vi "Actor Core.vi"(8 "error in":errorcluster, 11 "CS++GUIActor in":refnum<class "CS++GUIActor.lvclass">) -> (0 "error out":errorcluster, 3 "Actor out":refnum<class "Actor.lvclass">)   [LabVIEW 2013, in "CS++GUIActor.lvlib" / "CS++GUIActor.lvclass"]
doc: "(<B>Filename</B>: Actor Framework.lvlib:Actor.lvclass:Actor Core.vi)\n\nReceives messages to the actor, reacts to them, and initiates any error handling that may shut the actor down.\n\nDescendant classes may override this VI to append parallel tasks for the actor to complete while it handles messages. Overrides use the Call Parent Method node."
uses:
  CS++GUIActor.lvclass
  <vilib>/ActorFramework/Actor/Actor.lvclass
  CS++BaseActor/CS++BaseActor.lvclass/CS++BaseActor.ctl
  CS++GUIActor.lvclass/CS++GUIActor.ctl
  Classes/CS++BaseClasses/Factory/CS++Factory.lvclass
  CS++BaseActor/CS++BaseActor.lvclass
  <vilib>/ActorFramework/Actor/Actor.lvclass/Actor.ctl
  <vilib>/ActorFramework/Message Enqueuer/Message Enqueuer.lvclass/Message Enqueuer.ctl
  <vilib>/ActorFramework/Message Enqueuer/Init from Existing Queue.vi
  <vilib>/ActorFramework/Message Enqueuer/Enqueue.vi
  <vilib>/ActorFramework/Message Priority Queue/Priority Enqueue.vi
  <vilib>/ActorFramework/Message Enqueuer/Message Enqueuer.lvclass
  <vilib>/ActorFramework/Stop Msg/Stop Msg.lvclass
panel:
  in  "Stop Button":bool
  out "Actor Name":string
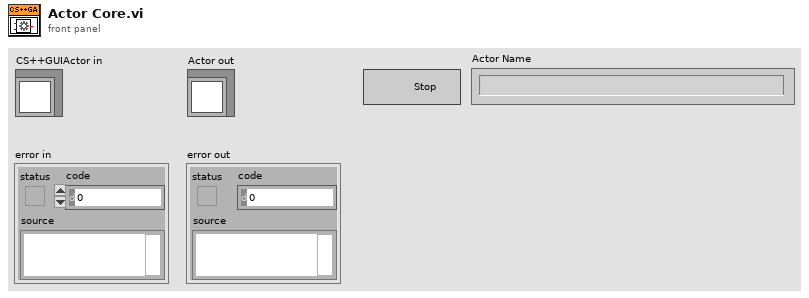
[diagram p1: front panel]
types:
  T1 = enum32{"Invalid", "Standard", "Closed", "Hidden", "Minimized", "Maximized"}
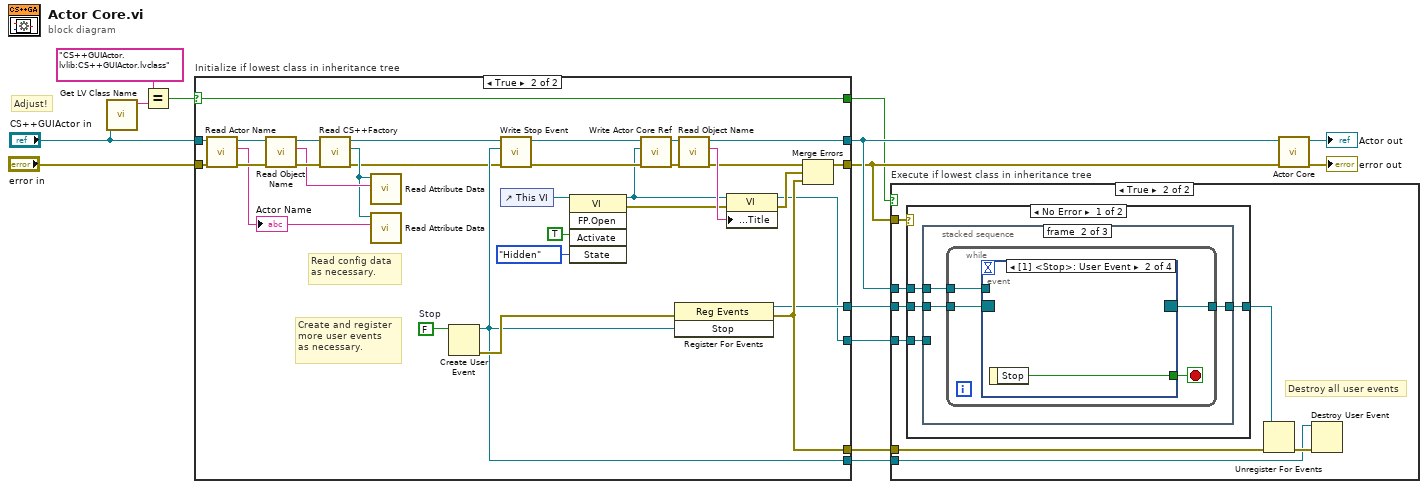
[diagram p0: block diagram]
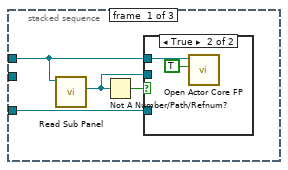
[diagram p3: hidden frame]
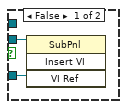
[diagram p4: hidden frame]
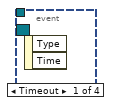
[diagram p5: hidden frame]
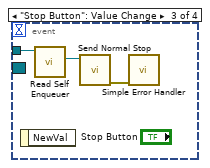
[diagram p6: hidden frame]
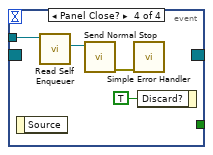
[diagram p7: hidden frame]
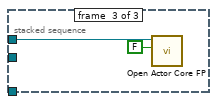
[diagram p8: hidden frame]
diagram:
  # "Adjust!"
  n1 = call <vilib>:"Get LV Class Name.vi"("object"="CS++GUIActor in") -> ("class name"=w13:string)  [unwired: 9 in, 1 out]
  n2 = Equal?(x="CS++GUIActor.lvlib:CS++GUIActor.lvclass" ("class name"), y=w13) -> (x = y?=w2:bool)
  n3 = case "Initialize if lowest class in inheritance tree" shown="True" w2 {
    selector: w2 -> [w17 w20]
    tunnel: "error in" -> [w15 w49]
    tunnel: "CS++GUIActor in" -> [w16 w48]
    tunnel: [_ w40] -> w8
    tunnel: [_ w39] -> w7
    tunnel: [_ w18] -> w6
    tunnel: [_ w30] -> w5
    tunnel: [w16 w22] -> w4
    tunnel: [w15 w21] -> w3
    tunnel: [w17 w20] -> w1
    frame False {
    }
    frame True {
      w43 = FALSE  # Stop
      # "Create and register \nmore user events\nas necessary."
      # "Read config data\nas necessary."
      n4 = call "Read Actor Name.vi"("error in (no error)"=w49, "CS++GUIActor in"=w48) -> ("error out"=w33:errorcluster, "Actor Name"=w31:string, "CS++GUIActor out"=w34:refnum<class "CS++GUIActor.lvclass">)  [unwired: 7 in]
      "Actor Name" <- w31
      n5 = call "Read Object Name.vi"("error in (no error)"=w33, "CS++BaseActor in"=w34) -> ("error out"=w36:errorcluster, "Object Name"=w35:string, "CS++BaseActor out"=w37:refnum<class "CS++GUIActor.lvclass">)  [unwired: 7 in]
      n6 = call "Read CS++Factory.vi"("error in (no error)"=w36, "CS++BaseActor in"=w37) -> ("error out"=w28:errorcluster, "CS++Factory"=w32:refnum<class "CS++Factory.lvclass">, "CS++BaseActor out"=w29:refnum<class "CS++GUIActor.lvclass">)  [unwired: 7 in]
      n7 = call-dynamic "Read Attribute Data.vi"("Object Name"=w35, "CS++Factory in"=w32) -> ()  [unwired: 7 in, 3 out]
      n8 = call-dynamic "Read Attribute Data.vi"("Object Name"=w31, "CS++Factory in"=w32) -> ()  [unwired: 7 in, 3 out]
      n9 = Create User Event(user event datatype=w43) -> (user event=w30:refnum<user-event>, error out=w41:errorcluster)  [unwired: 1 in]
      n10 = call "Write Stop Event.vi"("error in (no error)"=w28, "Stop"=w30, "CS++GUIActor in"=w29) -> ("error out"=w26:errorcluster, "CS++GUIActor out"=w27:refnum<class "CS++GUIActor.lvclass">)  [unwired: 7 in]
      n11 = control-ref of="This VI"() -> (w47:refnum<vi>)
      n12 = invoke class="VI" method="FP.Open"(reference=w47, "Activate"=TRUE ("Activate?"), "State"=T1."Hidden") -> (reference out=w19:refnum<vi>, error out=w38:errorcluster)  [unwired: 2 in, 3 out]
      n13 = call "Write Actor Core Ref.vi"("error in (no error)"=w26, "Actor Core Ref"=w19, "CS++BaseActor in"=w27) -> ("error out"=w25:errorcluster, "CS++BaseActor out"=w24:refnum<class "CS++GUIActor.lvclass">)  [unwired: 7 in]
      n14 = register-events(error in=w41, w30) -> (reference out=w39:refnum<event-registration>, error out=w40:errorcluster)  [unwired: 1 in]
      n15 = call "Read Object Name.vi"("error in (no error)"=w25, "CS++BaseActor in"=w24) -> ("error out"=w23:errorcluster, "Object Name"=w44:string, "CS++BaseActor out"=w22:refnum<class "CS++GUIActor.lvclass">)  [unwired: 7 in]
      n16 = property class="VI"(reference=w19, error in=w38, "Front Panel.Title"=w44) -> (reference out=w18:refnum<vi>, error out=w42:errorcluster)
      n17 = Merge Errors(w23, w42, w40) -> (w21:errorcluster)
    }
  }
  n18 = case "Execute if lowest class in inheritance tree" shown="True" w1 {
    tunnel: w8 -> [_ w56]
    tunnel: w7 -> [_ w55]
    tunnel: w6 -> [_ w53]
    tunnel: w5 -> [_ w52]
    tunnel: w4 -> [_ w51]
    tunnel: w3 -> [_ w50]
    frame False {
    }
    frame True {
      # "Destroy all user events"
      n19 = case shown="No Error" w50 {
        tunnel: w51 -> [w61 _]
        tunnel: w55 -> [w60 w87]
        tunnel: [w59 w87] -> w54
        tunnel: w53 -> [w58 _]
        frame No Error {
          n20 = stacked-sequence {
            tunnel: w61 -> [w63 w71 w86]
            tunnel: w60 -> [_ w72 _]
            tunnel: [_ w70 _] -> w59
            tunnel: w58 -> [w64 _ _]
            frame #0 {
              n21 = call "Read Sub Panel.vi"("CS++GUIActor in"=w63) -> ("Sub Panel"=w62:refnum<vi>)  [unwired: 8 in, 2 out]
              n22 = Not A Number/Path/Refnum?(number/path/refnum=w62) -> (NaN/Path/Refnum?=w65:bool)
              n23 = case shown="True" w65 {
                tunnel: w63 -> [_ w69]
                tunnel: w62 -> [w67 _]
                tunnel: w64 -> [w66 _]
                frame False {
                  n24 = invoke class="SubPnl" method="Insert VI"(reference=w67, "VI Ref"=w66) -> ()  [unwired: 2 in, 4 out]
                }
                frame True {
                  n25 = call "Open Actor Core FP.vi"("Open FP (F)"=TRUE, "CS++BaseActor in"=w69) -> ()  [unwired: 8 in, 2 out]
                }
              }
            }
            frame #1 {
              n26 = while {
                tunnel: w72 -> [w76]
                tunnel: w71 -> [w75]
                tunnel: [w73] -> w70
                stop <- w74 stop-if-true
                n27 = event shown="[1] <Stop>: User Event" {
                  selector: w76 -> [_ _ _ _]
                  dyn-events: [_ _ _ _] -> w73
                  timeout: _ -> [_ _ _ _]
                  tunnel: w75 -> [_ _ w80 w81]
                  tunnel: [_ w77 _ _] -> w74
                  event Timeout {
                    n28 = event-data() -> ()  [unwired: 1 in, 2 out]
                  }
                  event User Event {
                    n29 = event-data() -> ("Stop"=w77:bool)  [unwired: 1 in]
                  }
                  event "Stop Button": Value Change {
                    n30 = event-data() -> ()  [unwired: 1 in, 1 out]
                    n31 = call <vilib>:"Read Self Enqueuer.vi"("Actor"=w80) -> ("Self Enqueuer"=w79:refnum<class "Message Enqueuer.lvclass">)  [unwired: 10 in]
                    n32 = call <vilib>:"Send Normal Stop.vi"("Message Enqueuer"=w79) -> ("error out"=w78:errorcluster)  [unwired: 10 in]
                    n33 = call <vilib>:"Simple Error Handler.vi"("error in (no error)"=w78) -> ()  [unwired: 4 in, 5 out]
                  }
                  event Panel Close? {
                    n34 = event-data() -> ()  [unwired: 1 in, 1 out]
                    n35 = call <vilib>:"Read Self Enqueuer.vi"("Actor"=w81) -> ("Self Enqueuer"=w83:refnum<class "Message Enqueuer.lvclass">)  [unwired: 10 in]
                    n36 = call <vilib>:"Send Normal Stop.vi"("Message Enqueuer"=w83) -> ("error out"=w82:errorcluster)  [unwired: 10 in]
                    n37 = call <vilib>:"Simple Error Handler.vi"("error in (no error)"=w82) -> ()  [unwired: 4 in, 5 out]
                    n38 = event-data("Discard?"=TRUE) -> ()  [unwired: 1 in, 1 out]
                  }
                }
              }
            }
            frame #2 {
              n39 = call "Open Actor Core FP.vi"("Open FP (F)"=FALSE, "CS++BaseActor in"=w86) -> ()  [unwired: 8 in, 2 out]
            }
          }
        }
        frame Error {
        }
      }
      n40 = Unregister For Events(event registration refnum=w54, error in=w56) -> (error out=w57:errorcluster)
      n41 = Destroy User Event(user event=w52, error in=w57) -> ()  [unwired: 1 out]
    }
  }
  n42 = call-parent "Actor Core.vi"("error in"=w3, "CS++BaseActor in"=w4) -> ("error out"=→"error out":errorcluster, "Actor out"=→"Actor out":refnum<class "Actor.lvclass">)  [unwired: 8 in]
